vi "Traffic Light task.vi"() -> ()   [LabVIEW 2016]
panel:
  out "South Bound Left":T1
  out "South Bound":T1={"R"=TRUE, "Y"=FALSE, "G"=FALSE, "Elapsed"=0}
  out "West Bound Left":T1
  out "West Bound":T1={"R"=TRUE, "Y"=FALSE, "G"=FALSE, "Elapsed"=0}
  out "East Bound Left":T1
  out "East Bound":T1={"R"=TRUE, "Y"=FALSE, "G"=FALSE, "Elapsed"=0}
  out "North Bound Left":T1
  out "North Bound":T1={"R"=TRUE, "Y"=FALSE, "G"=FALSE, "Elapsed"=0}
  in  "Cluster":T2
  in  "North  Sensor  2":bool
  in  "West Sensor 2":bool
  in  "East Sensor 2":bool
  in  "South Sensor 2":bool
  in  "stop 2":bool
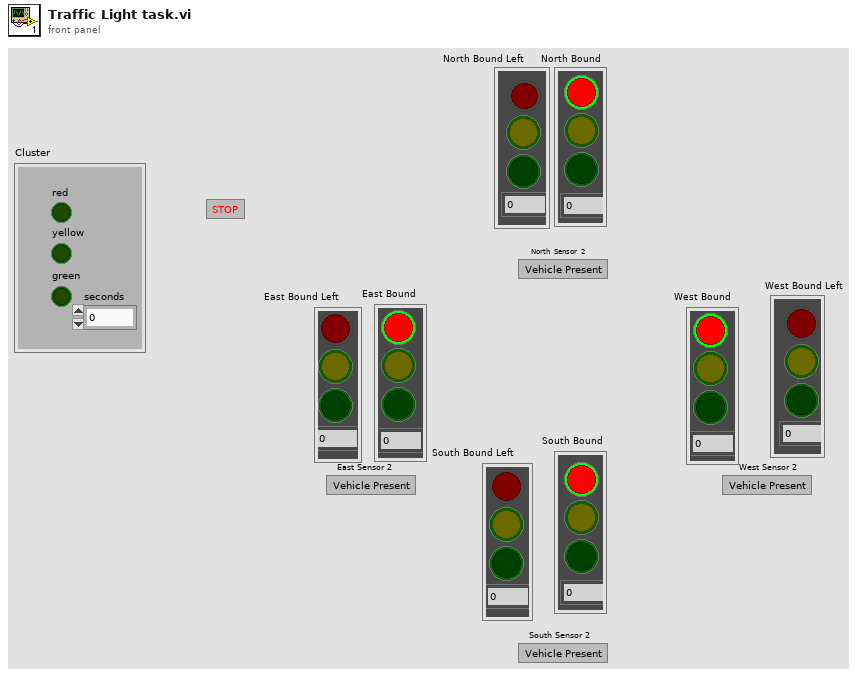
[diagram p1: front panel]
types:
  T1 = cluster{"R":bool, "Y":bool, "G":bool, "Elapsed":u32}
  T2 = cluster{"red":bool, "yellow":bool, "green":bool, "seconds":dbl}
  T3 = enum16{"ns green", "ns yellow", "ns red", "ew green", "ew yellow", "ew red", "nsl green", "ewl green"}
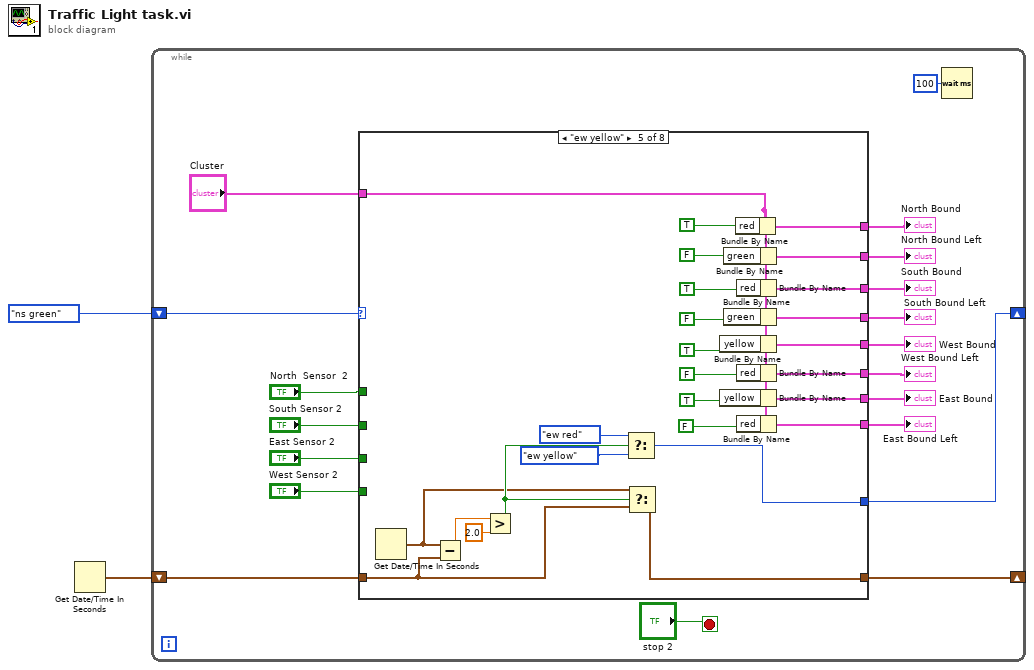
[diagram p0: block diagram]
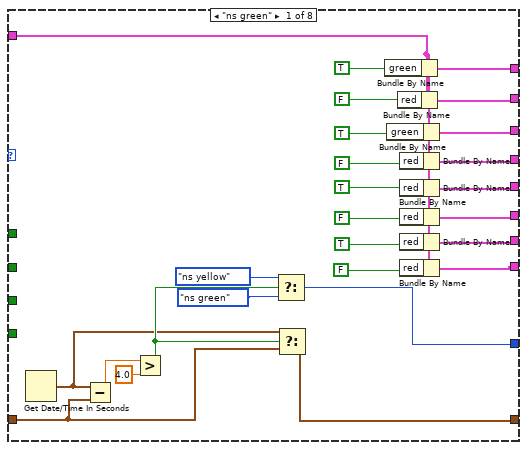
[diagram p2: hidden frame]
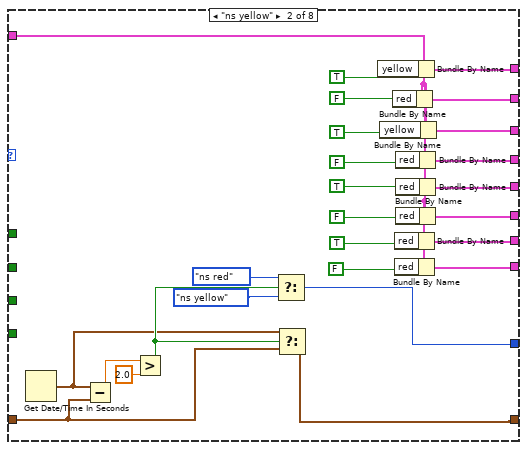
[diagram p3: hidden frame]
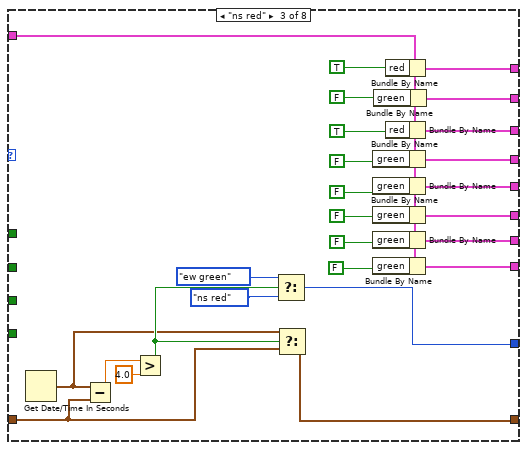
[diagram p4: hidden frame]
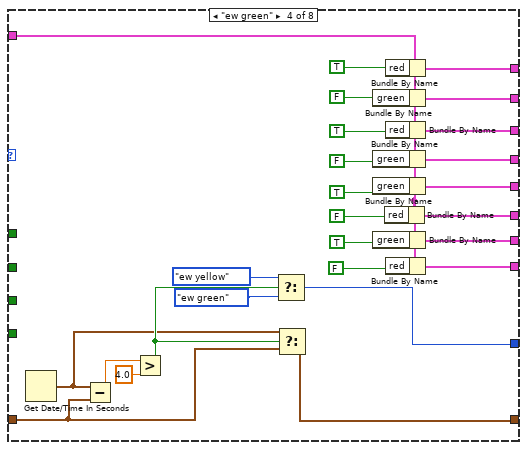
[diagram p5: hidden frame]
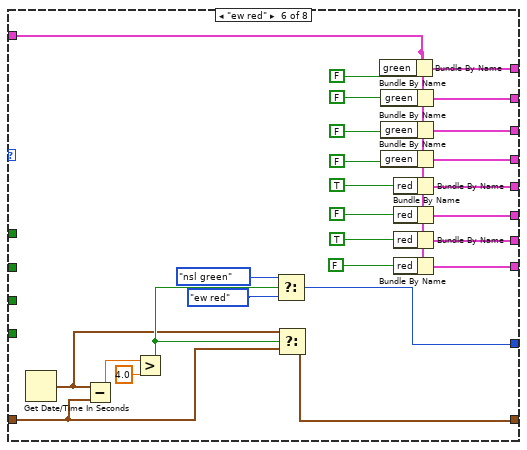
[diagram p6: hidden frame]
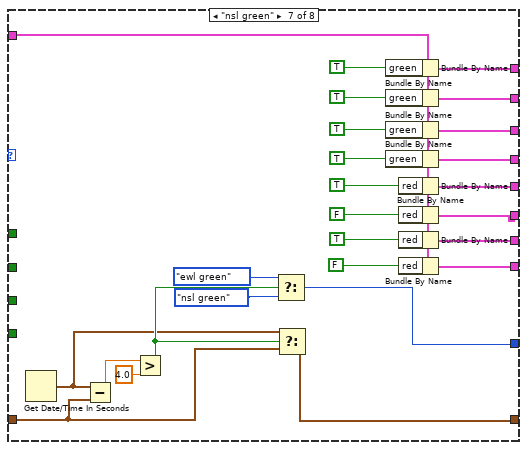
[diagram p7: hidden frame]
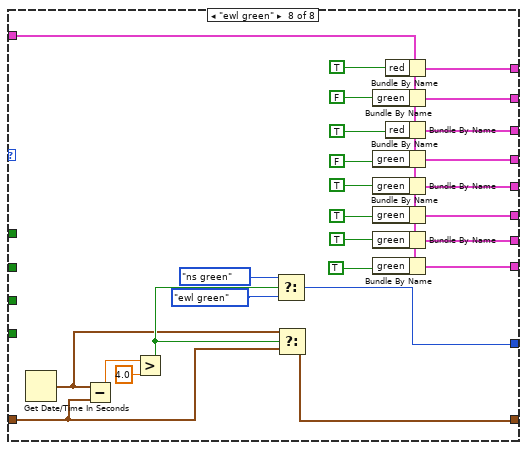
[diagram p8: hidden frame]
diagram:
  n1 = Get Date/Time In Seconds() -> (seconds since 1Jan1904=w2:timestamp)
  n2 = while {
    shift-right: [w4] -> _
    shift-left: w2 -> [w16]
    shift-right: [w3] -> _
    shift-left: T3."ns green" ("Enum") -> [w12]
    stop <- "stop 2" stop-if-true
    n3 = case shown="\"ew yellow\"" w12 {
      tunnel: "North  Sensor  2" -> [_ _ _ _ _ _ _ _]
      tunnel: "South Sensor 2" -> [_ _ _ _ _ _ _ _]
      tunnel: "East Sensor 2" -> [_ _ _ _ _ _ _ _]
      tunnel: "West Sensor 2" -> [_ _ _ _ _ _ _ _]
      tunnel: w16 -> [w37 w64 w89 w115 w141 w167 w195 w219]
      tunnel: [w43 w70 w95 w121 w147 w173 w200 w225] -> w3
      tunnel: [w44 w48 w96 w122 w148 w174 w187 w226] -> w4
      tunnel: [w42 w69 w94 w120 w146 w172 w185 w224] -> w14
      tunnel: "Cluster" -> [w30 w56 w81 w107 w133 w159 w186 w211]
      tunnel: [w29 w55 w80 w106 w132 w158 w184 w210] -> w11
      tunnel: [w28 w54 w79 w105 w131 w157 w183 w209] -> w10
      tunnel: [w27 w53 w78 w104 w130 w156 w182 w208] -> w9
      tunnel: [w26 w52 w77 w103 w129 w155 w181 w207] -> w8
      tunnel: [w25 w51 w76 w102 w128 w154 w180 w206] -> w7
      tunnel: [w24 w50 w75 w101 w127 w153 w179 w205] -> w6
      tunnel: [w23 w49 w74 w100 w126 w152 w178 w204] -> w5
      frame "ns green" {
        n4 = Get Date/Time In Seconds() -> (seconds since 1Jan1904=w36:timestamp)
        n5 = Subtract(x=w36, y=w37) -> (x-y=w46:dbl)
        n6 = Greater?(x=w46, y=4.0) -> (0:w45:bool)
        n7 = Select(t=T3."ns yellow" ("Enum"), s=w45, f=T3."ns green" ("Enum")) -> (s? t:f=w43:T3)
        n8 = Select(t=w36, s=w45, f=w37) -> (s? t:f=w44:timestamp)
        n9 = Bundle By Name(cluster=w30, "green"=TRUE) -> (w42:T2)
        n10 = Bundle By Name(cluster=w30, "green"=TRUE) -> (w28:T2)
        n11 = Bundle By Name(cluster=w30, "red"=FALSE ("green")) -> (w29:T2)
        n12 = Bundle By Name(cluster=w30, "red"=FALSE ("green")) -> (w27:T2)
        n13 = Bundle By Name(cluster=w30, "red"=TRUE ("green")) -> (w26:T2)
        n14 = Bundle By Name(cluster=w30, "red"=FALSE ("green")) -> (w25:T2)
        n15 = Bundle By Name(cluster=w30, "red"=TRUE ("green")) -> (w24:T2)
        n16 = Bundle By Name(cluster=w30, "red"=FALSE ("green")) -> (w23:T2)
      }
      frame "ns yellow" {
        n17 = Get Date/Time In Seconds() -> (seconds since 1Jan1904=w63:timestamp)
        n18 = Subtract(x=w63, y=w64) -> (x-y=w72:dbl)
        n19 = Greater?(x=w72, y=2.0) -> (0:w71:bool)
        n20 = Select(t=T3."ns red" ("Enum"), s=w71, f=T3."ns yellow" ("Enum")) -> (s? t:f=w70:T3)
        n21 = Select(t=w63, s=w71, f=w64) -> (s? t:f=w48:timestamp)
        n22 = Bundle By Name(cluster=w56, "yellow"=TRUE) -> (w69:T2)
        n23 = Bundle By Name(cluster=w56, "yellow"=TRUE ("green")) -> (w54:T2)
        n24 = Bundle By Name(cluster=w56, "red"=FALSE ("green")) -> (w55:T2)
        n25 = Bundle By Name(cluster=w56, "red"=TRUE ("green")) -> (w50:T2)
        n26 = Bundle By Name(cluster=w56, "red"=FALSE ("green")) -> (w49:T2)
        n27 = Bundle By Name(cluster=w56, "red"=FALSE ("green")) -> (w53:T2)
        n28 = Bundle By Name(cluster=w56, "red"=TRUE ("green")) -> (w52:T2)
        n29 = Bundle By Name(cluster=w56, "red"=FALSE ("green")) -> (w51:T2)
      }
      frame "ns red" {
        n30 = Get Date/Time In Seconds() -> (seconds since 1Jan1904=w88:timestamp)
        n31 = Subtract(x=w88, y=w89) -> (x-y=w98:dbl)
        n32 = Greater?(x=w98, y=4.0) -> (0:w97:bool)
        n33 = Select(t=T3."ew green" ("Enum"), s=w97, f=T3."ns red" ("Enum")) -> (s? t:f=w95:T3)
        n34 = Select(t=w88, s=w97, f=w89) -> (s? t:f=w96:timestamp)
        n35 = Bundle By Name(cluster=w81, "green"=FALSE) -> (w78:T2)
        n36 = Bundle By Name(cluster=w81, "green"=FALSE) -> (w77:T2)
        n37 = Bundle By Name(cluster=w81, "green"=FALSE) -> (w76:T2)
        n38 = Bundle By Name(cluster=w81, "green"=FALSE) -> (w75:T2)
        n39 = Bundle By Name(cluster=w81, "green"=FALSE) -> (w74:T2)
        n40 = Bundle By Name(cluster=w81, "green"=FALSE) -> (w80:T2)
        n41 = Bundle By Name(cluster=w81, "red"=TRUE) -> (w94:T2)
        n42 = Bundle By Name(cluster=w81, "red"=TRUE ("green")) -> (w79:T2)
      }
      frame "ew green" {
        n43 = Get Date/Time In Seconds() -> (seconds since 1Jan1904=w114:timestamp)
        n44 = Subtract(x=w114, y=w115) -> (x-y=w124:dbl)
        n45 = Greater?(x=w124, y=4.0) -> (0:w123:bool)
        n46 = Select(t=T3."ew yellow" ("Enum"), s=w123, f=T3."ew green" ("Enum")) -> (s? t:f=w121:T3)
        n47 = Select(t=w114, s=w123, f=w115) -> (s? t:f=w122:timestamp)
        n48 = Bundle By Name(cluster=w107, "green"=FALSE) -> (w106:T2)
        n49 = Bundle By Name(cluster=w107, "green"=FALSE) -> (w104:T2)
        n50 = Bundle By Name(cluster=w107, "green"=TRUE) -> (w103:T2)
        n51 = Bundle By Name(cluster=w107, "green"=TRUE) -> (w101:T2)
        n52 = Bundle By Name(cluster=w107, "red"=FALSE ("green")) -> (w102:T2)
        n53 = Bundle By Name(cluster=w107, "red"=TRUE) -> (w120:T2)
        n54 = Bundle By Name(cluster=w107, "red"=TRUE ("green")) -> (w105:T2)
        n55 = Bundle By Name(cluster=w107, "red"=FALSE ("green")) -> (w100:T2)
      }
      frame "ew yellow" {
        n56 = Get Date/Time In Seconds() -> (seconds since 1Jan1904=w140:timestamp)
        n57 = Subtract(x=w140, y=w141) -> (x-y=w150:dbl)
        n58 = Greater?(x=w150, y=2.0) -> (0:w149:bool)
        n59 = Select(t=T3."ew red" ("Enum"), s=w149, f=T3."ew yellow" ("Enum")) -> (s? t:f=w147:T3)
        n60 = Select(t=w140, s=w149, f=w141) -> (s? t:f=w148:timestamp)
        n61 = Bundle By Name(cluster=w133, "yellow"=TRUE ("green")) -> (w129:T2)
        n62 = Bundle By Name(cluster=w133, "yellow"=TRUE ("green")) -> (w127:T2)
        n63 = Bundle By Name(cluster=w133, "green"=FALSE) -> (w132:T2)
        n64 = Bundle By Name(cluster=w133, "green"=FALSE) -> (w130:T2)
        n65 = Bundle By Name(cluster=w133, "red"=TRUE) -> (w146:T2)
        n66 = Bundle By Name(cluster=w133, "red"=TRUE ("green")) -> (w131:T2)
        n67 = Bundle By Name(cluster=w133, "red"=FALSE ("green")) -> (w128:T2)
        n68 = Bundle By Name(cluster=w133, "red"=FALSE ("green")) -> (w126:T2)
      }
      frame "ew red" {
        n69 = Get Date/Time In Seconds() -> (seconds since 1Jan1904=w166:timestamp)
        n70 = Subtract(x=w166, y=w167) -> (x-y=w176:dbl)
        n71 = Greater?(x=w176, y=4.0) -> (0:w175:bool)
        n72 = Select(t=T3."nsl green" ("Enum"), s=w175, f=T3."ew red" ("Enum")) -> (s? t:f=w173:T3)
        n73 = Select(t=w166, s=w175, f=w167) -> (s? t:f=w174:timestamp)
        n74 = Bundle By Name(cluster=w159, "green"=FALSE) -> (w172:T2)
        n75 = Bundle By Name(cluster=w159, "green"=FALSE) -> (w158:T2)
        n76 = Bundle By Name(cluster=w159, "green"=FALSE) -> (w157:T2)
        n77 = Bundle By Name(cluster=w159, "green"=FALSE) -> (w156:T2)
        n78 = Bundle By Name(cluster=w159, "red"=TRUE ("green")) -> (w155:T2)
        n79 = Bundle By Name(cluster=w159, "red"=FALSE ("green")) -> (w154:T2)
        n80 = Bundle By Name(cluster=w159, "red"=TRUE ("green")) -> (w153:T2)
        n81 = Bundle By Name(cluster=w159, "red"=FALSE ("green")) -> (w152:T2)
      }
      frame "nsl green" {
        n82 = Get Date/Time In Seconds() -> (seconds since 1Jan1904=w194:timestamp)
        n83 = Subtract(x=w194, y=w195) -> (x-y=w202:dbl)
        n84 = Greater?(x=w202, y=4.0) -> (0:w201:bool)
        n85 = Select(t=T3."ewl green" ("Enum"), s=w201, f=T3."nsl green" ("Enum")) -> (s? t:f=w200:T3)
        n86 = Select(t=w194, s=w201, f=w195) -> (s? t:f=w187:timestamp)
        n87 = Bundle By Name(cluster=w186, "green"=TRUE) -> (w185:T2)
        n88 = Bundle By Name(cluster=w186, "green"=TRUE) -> (w184:T2)
        n89 = Bundle By Name(cluster=w186, "green"=TRUE) -> (w183:T2)
        n90 = Bundle By Name(cluster=w186, "green"=TRUE) -> (w182:T2)
        n91 = Bundle By Name(cluster=w186, "red"=TRUE ("green")) -> (w181:T2)
        n92 = Bundle By Name(cluster=w186, "red"=FALSE ("green")) -> (w180:T2)
        n93 = Bundle By Name(cluster=w186, "red"=TRUE ("green")) -> (w179:T2)
        n94 = Bundle By Name(cluster=w186, "red"=FALSE ("green")) -> (w178:T2)
      }
      frame "ewl green" {
        n95 = Get Date/Time In Seconds() -> (seconds since 1Jan1904=w218:timestamp)
        n96 = Subtract(x=w218, y=w219) -> (x-y=w228:dbl)
        n97 = Greater?(x=w228, y=4.0) -> (0:w227:bool)
        n98 = Select(t=T3."ns green" ("Enum"), s=w227, f=T3."ewl green" ("Enum")) -> (s? t:f=w225:T3)
        n99 = Select(t=w218, s=w227, f=w219) -> (s? t:f=w226:timestamp)
        n100 = Bundle By Name(cluster=w211, "green"=FALSE) -> (w210:T2)
        n101 = Bundle By Name(cluster=w211, "green"=FALSE) -> (w208:T2)
        n102 = Bundle By Name(cluster=w211, "green"=TRUE) -> (w207:T2)
        n103 = Bundle By Name(cluster=w211, "green"=TRUE) -> (w206:T2)
        n104 = Bundle By Name(cluster=w211, "green"=TRUE) -> (w205:T2)
        n105 = Bundle By Name(cluster=w211, "green"=TRUE) -> (w204:T2)
        n106 = Bundle By Name(cluster=w211, "red"=TRUE) -> (w224:T2)
        n107 = Bundle By Name(cluster=w211, "red"=TRUE ("green")) -> (w209:T2)
      }
    }
    "North Bound" <- w14
    "North Bound Left" <- w11
    "East Bound" <- w6
    "East Bound Left" <- w5
    "West Bound" <- w8
    "West Bound Left" <- w7
    "South Bound" <- w10
    "South Bound Left" <- w9
    n108 = Wait (ms)(milliseconds to wait=u32 100) -> ()  [unwired: 1 out]
  }
